vi "Auto Intake.vi"(10 "Intake Commands":T1, 11 "Intake Mode":T2) -> (3 "isFinished":bool)   [LabVIEW 2015]
uses:
  Common Code/Intake Mode.ctl
  Common Code/Intake Commands.ctl
  Robot Global Data.vi
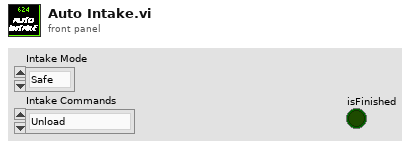
[diagram p1: front panel]
types:
  T1 = typedef "Intake Commands.ctl" = enum16{"Unload", "Load", "Pull up", "Drop low", "Idle", "Lift Half"}
  T2 = typedef "Intake Mode.ctl" = enum16{"Safe", "Auto", "Manual"}
  T3 = typedef "Intake Status Cluster.ctl" = cluster{"Roller Power":dbl, "Angle Power":dbl, "Intake Mode":T2, "Intake States":T4, "Rollers Active?":bool, "Height":dbl, "Intake Encoder Cluster":T5}
  T4 = typedef "Intake States.ctl" = enum16{"Idle", "Set roller speed", "Move to angle"}
  T5 = typedef "IntakeEncoderCluster.ctl" = cluster{"Arm Motor Encoder Values":cluster{"Ticks":dbl, "Speed":dbl, "Distance":dbl}}
  T6 = typedef "Intake Commands Cluster.ctl" = cluster{"Intake Commands":T1, "Intake Mode":T2, "Encoder Constraint":dbl}
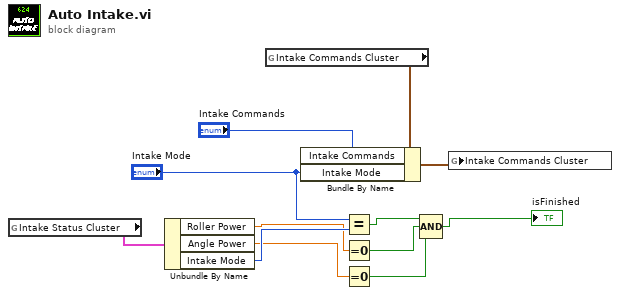
[diagram p0: block diagram]
diagram:
  n1 = global read "Robot Global Data.vi" "Intake Status Cluster"() -> (w9:T3)
  n2 = Unbundle By Name(w9) -> ("Roller Power"=w6:dbl, "Angle Power"=w5:dbl, "Intake Mode"=w7:T2)
  n3 = global read "Robot Global Data.vi" "Intake Commands Cluster"() -> (w11:T6)
  n4 = Bundle By Name(cluster=w11, "Intake Commands"="Intake Commands", "Intake Mode"="Intake Mode") -> (w12:T6)
  n5 = Equal?(x="Intake Mode", y=w7) -> (x = y?=w4:bool)
  n6 = Equal To 0?(x=w6) -> (x = 0?=w3:bool)
  n7 = Equal To 0?(x=w5) -> (x = 0?=w2:bool)
  n8 = Compound Arithmetic op=AND(w4, w3, w2) -> (→"isFinished":bool)
  n9 = global write "Robot Global Data.vi" "Intake Commands Cluster"(w12) -> ()
